vi "Set Compiled Code Option.vi"(8 "error in (no error)":errorcluster, 10 "Compiled code option":T1, 11 "NI_AB_API_SDIST in":refnum<class "NI_AB_API_SDIST.lvclass">) -> (0 "error out":errorcluster, 3 "NI_AB_API_SDIST out":refnum<class "NI_AB_API_SDIST.lvclass">)   [LabVIEW 2020, in "NI_AB_API_SDIST.lvclass"]
uses:
  <vilib>/AppBuilder/AB_API/SDIST/NI_AB_API_SDIST.lvclass
  <vilib>/AppBuilder/AB_API/SDIST/NI_AB_API_SDIST.lvclass/NI_AB_API_SDIST.ctl
  <vilib>/AppBuilder/AB_Classes/Build/AB_Build.lvclass
  <vilib>/AppBuilder/AB_API/Build/NI_AB_API_Build.lvclass
  e:/builds/penguin/labview/branches/2020/dev/dist/vi.lib/AppBuilder/AB_API/Build/NI_AB_API_Build.lvclass
  e:/builds/penguin/labview/branches/2020/dev/dist/vi.lib/AppBuilder/AB_API/SDIST/NI_AB_API_SDIST.lvclass
  <vilib>/AppBuilder/AB_API/common/AB_API Compiled Code Option.ctl
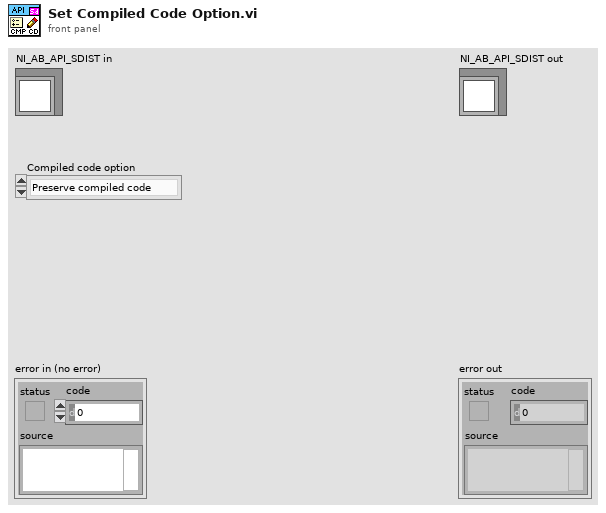
[diagram p1: front panel]
types:
  T1 = typedef "AB_API Compiled Code Option.ctl" = enum16{"Preserve compiled code", "Remove compiled code", "Preserve file settings"}
  T2 = typedef "AB_Build.ctl" = cluster{"buildSpecName":string, "buildSpecDescription":string, "destinations":refnum<class "AB_Destination.lvclass">[], "exclusionOption":T3, "defaultLanguage":string, "supportedLanguages":string[], "excludedDirectories":path[], "buildContext":refnum<vi>, "buildObject":T4, "preview":bool, "programatic":bool, "progressBarEvents":T5, "userLog_Path":path, "preActionID":string, "preAction_Path":path, "postActionID":string, "postAction_Path":path, "eng_checkForBrokenVIs?":bool, "eng_verboseLinkerErrors?":bool, "localDest_Path":path, "targetDest_Path":path, "removeVIObject":u16, "cache":refnum<class "PreviewCache.lvclass">, "use cache":bool, "previewCache_ID":string, "buildCache_ID":string, "eng_TempLocalDest_Path":path, "eng_collectDependencies?":bool, "versionInfo":cluster{"buildVersion":cluster{"major":u16, "minor":u16, "patch":u16, "build":u16}, "autoIncrement":bool}, "eng_enableVIChecksums":bool}
  T3 = typedef "AB_Exclusion_Option.ctl" = cluster{"typedefs":bool, "polymorphicVIs":bool, "unusedLibraryItems":bool, "modifyLibraryFile":bool, "edit-timeDependencies":bool, "inlineVIs":bool, "dependent PPLs":bool, "dependent DLLs":bool}
  T4 = typedef "ItemRef.ctl" = u64
  T5 = typedef "provcom_ProgressBar_Events.ctl" = cluster{"newJob":refnum<user-event>, "newItem":refnum<user-event>, "errorMsg":T6, "cancel":refnum<user-event>}
  T6 = typedef "mxLvBuildError.ctl" = refnum<user-event>
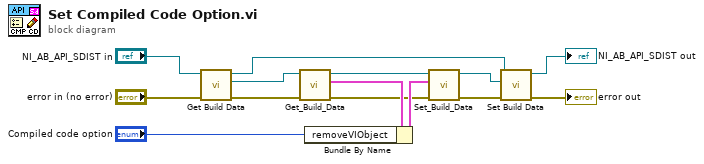
[diagram p0: block diagram]
diagram:
  n1 = call <vilib>:"Get Build Data.vi"("error in (no error)"="error in (no error)", "NI_AB_API_Build in"="NI_AB_API_SDIST in") -> ("error out"=w1:errorcluster, "AB_Build.lvclass"=w11:refnum<class "AB_Build.lvclass">, "NI_AB_API_Build out"=w9:refnum<class "NI_AB_API_SDIST.lvclass">)  [unwired: 7 in]
  n2 = call <vilib>:"Get_Build_Data.vi"("error in (no error)"=w1, "Class in"=w11) -> ("error out"=w5:errorcluster, "data"=w7:T2, "Class out"=w8:refnum<class "AB_Build.lvclass">)  [unwired: 7 out]
  n3 = Bundle By Name(cluster=w7, "removeVIObject"="Compiled code option") -> (w6:T2)
  n4 = call <vilib>:"Set_Build_Data.vi"("error in (no error)"=w5, "data"=w6, "Class in"=w8) -> ("error out"=w4:errorcluster, "Class out"=w10:refnum<class "AB_Build.lvclass">)  [unwired: 7 out]
  n5 = call <vilib>:"Set Build Data.vi"("error in (no error)"=w4, "AB_Build.lvclass"=w10, "NI_AB_API_Build in"=w9) -> ("error out"=→"error out":errorcluster, "NI_AB_API_Build out"=→"NI_AB_API_SDIST out":refnum<class "NI_AB_API_SDIST.lvclass">)  [unwired: 7 in]
